vi "Read Buffers.vi"(8 "error in (no error)":errorcluster, 11 "BufferMap in":refnum<data-value>) -> (0 "error out":errorcluster, 1 "Names":string[](array[string]), 2 "Buffers":refnum<data-value>[](array[refnum]), 3 "BufferMap":refnum<data-value>)   [LabVIEW 2013, in "VariantBufferMap.lvclass"]
uses:
  VariantBufferMap.lvclass
  VariantBuffer/VariantBuffer.lvclass
  VariantBufferMap.lvclass/VariantBufferMap.ctl
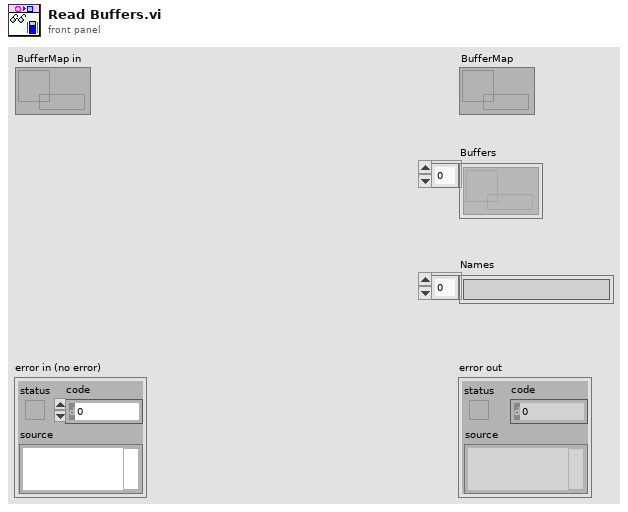
[diagram p1: front panel]
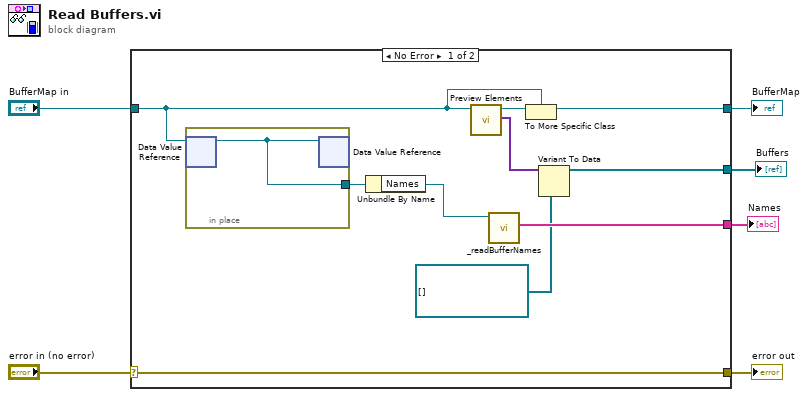
[diagram p0: block diagram]
diagram:
  n1 = case shown="No Error" "error in (no error)" {
    selector: "error in (no error)" -> [w16 w19]
    tunnel: [w16 w19] -> w5
    tunnel: [w13 w18] -> w3
    tunnel: "BufferMap in" -> [w12 w18]
    tunnel: [w10 _] -> w2
    tunnel: [w8 _] -> w1
    frame No Error {
      n2 = in-place {
        in-place-border: [w17] -> w15
        n3 = in-place-dvr #1(w12) -> (w17:refnum<class "VariantBufferMap.lvclass">)  [unwired: 1 out]
        n4 = in-place-dvr #1(w17) -> ()  [unwired: 2 out]
      }
      n5 = Unbundle By Name(w15) -> ("Names"=w11:refnum<data-value>)
      n6 = call "Preview Elements.vi"("ByteBuffer in"=w12) -> ("elements"=w9:variant[], "ByteBuffer"=w14:refnum<data-value>)  [unwired: 8 in, 1 out]
      n7 = call "_readBufferNames.vi"("Data Value Reference in"=w11) -> ("Names"=w10:string[])  [unwired: 9 in, 1 out]
      n8 = To More Specific Class(target class=w12, reference=w14) -> (specific class reference=w13:refnum<data-value>)  [unwired: 1 in, 1 out]
      n9 = Variant To Data(type=refnum<data-value>[] [] ("Buffers"), Variant=w9) -> (data=w8:refnum<data-value>[])  [unwired: 1 in, 1 out]
    }
    frame Error {
    }
  }
  "error out" <- w5
  "BufferMap" <- w3
  "Buffers" <- w1
  "Names" <- w2
